vi "Task Scheduler Test.vi"() -> ()   [LabVIEW 2015]
uses:
  Re-use Libraries/Minimal Actor Framework/Actors/Base Actor/Actor/Common Config.ctl
  Re-use Libraries/Minimal Actor Framework/Actors/Base Actor/Actor/Front Panel State.ctl
  Re-use Libraries/Minimal Actor Framework/Messaging/Messenger/Messenger.lvclass
  Globals.vi
  Actors/Task Scheduler/API/Task Scheduler Actor API.lvclass
  Re-use Libraries/Minimal Actor Framework/Actors/Base Actor/Actor/Actor.lvclass
  Actors/Task Scheduler/Actor/Task Scheduler Actor.lvclass
panel:
  in  "Log Name":string
  in  "Period 2":dbl
  in  "Period":dbl
  in  "Data Logging":bool
  in  "Heartbeat":bool
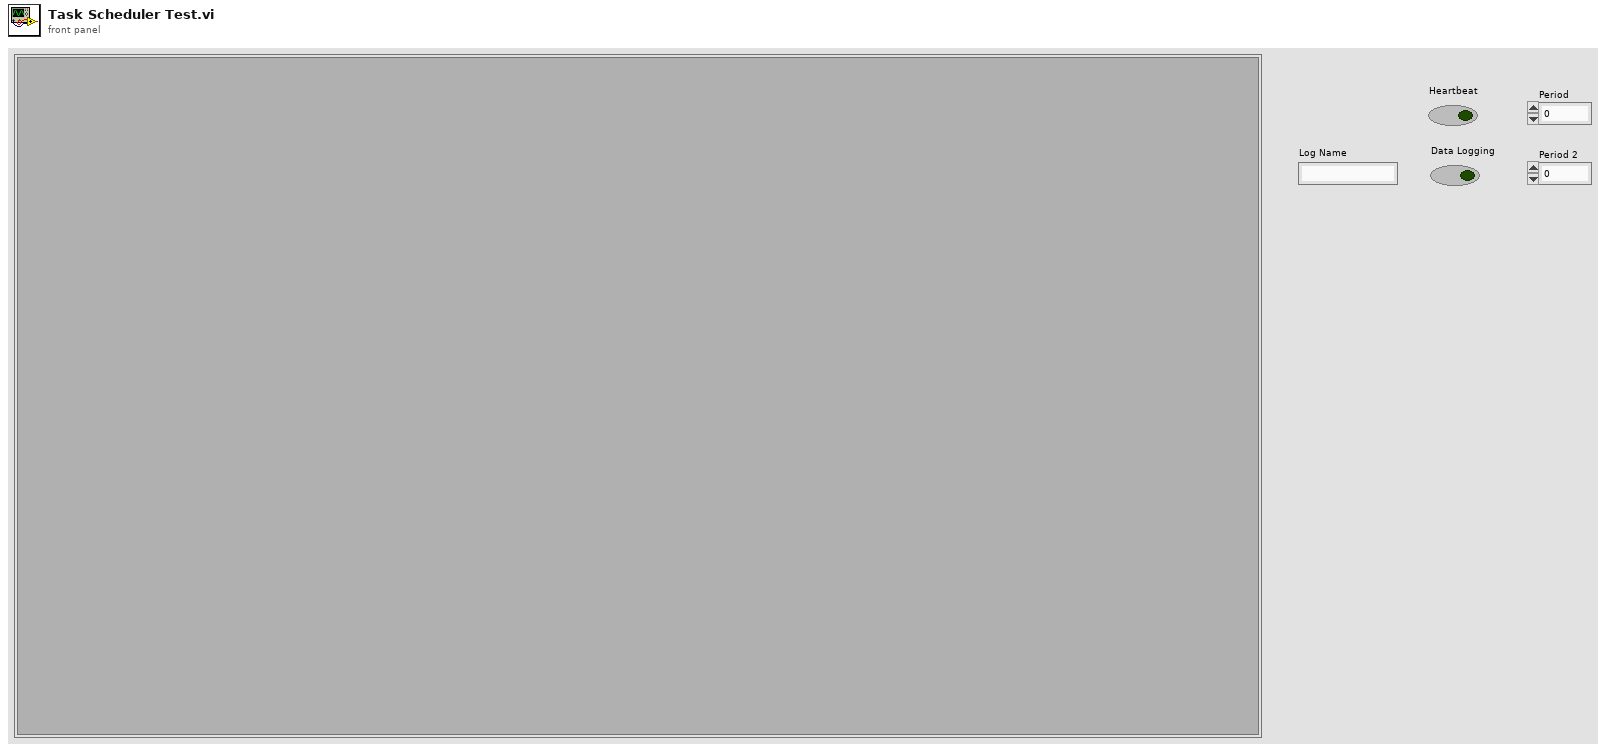
[diagram p1: front panel]
types:
  T1 = typedef "Actor.lvclass/Front Panel State.ctl" = enum32{"Invalid", "Standard", "Closed", "Hidden", "Minimized", "Maximized"}
  T2 = typedef "Actor.lvclass/Common Config.ctl" = cluster{"Launch Timeout [ms]":i32, "Wait For Launch Completed":bool, "Front Panel State":T1, "Close FP On Shutdown":bool, "Response Channel":refnum<class "Messenger.lvclass">, "Sub Panel":refnum<vi>}
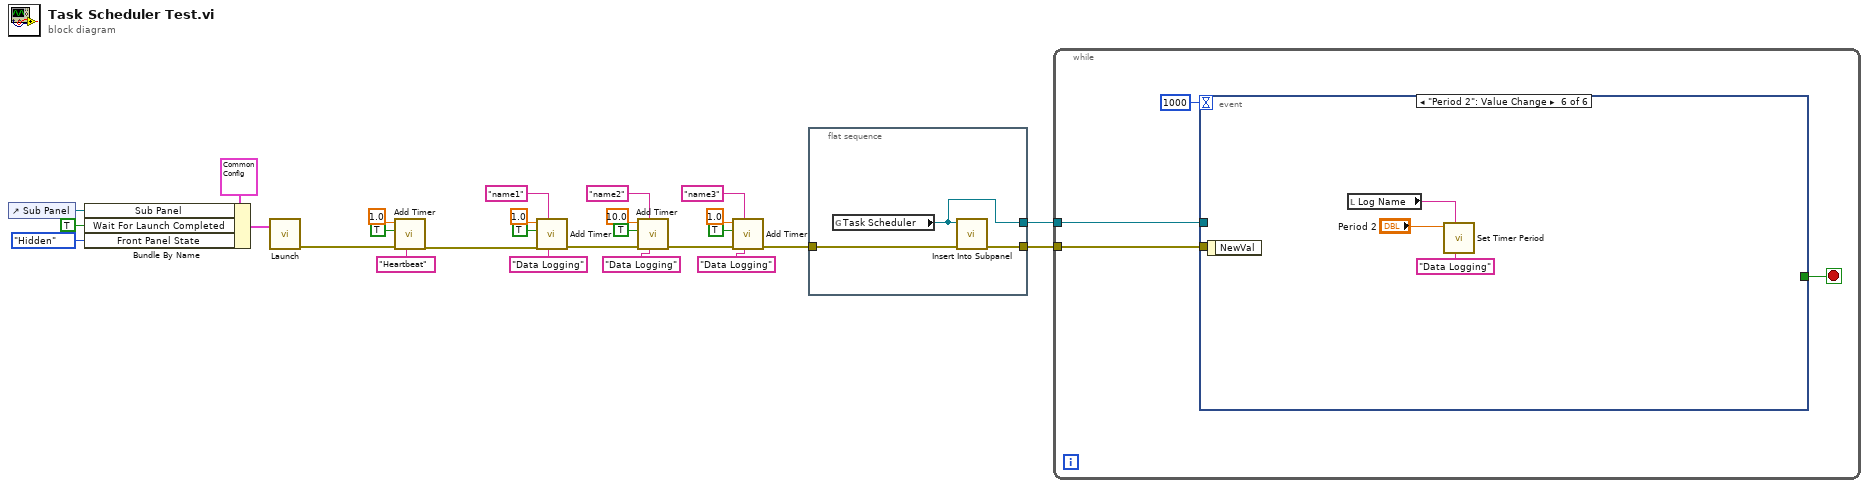
[diagram p0: block diagram]
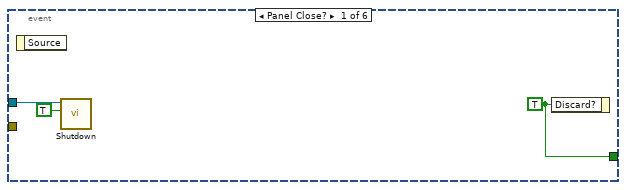
[diagram p2: hidden frame]
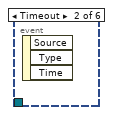
[diagram p3: hidden frame]
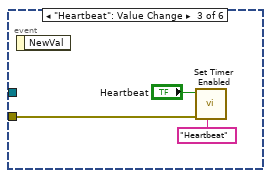
[diagram p4: hidden frame]
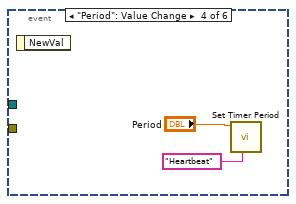
[diagram p5: hidden frame]
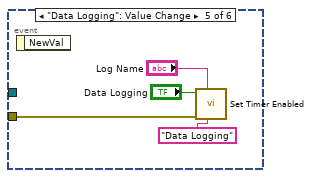
[diagram p6: hidden frame]
diagram:
  n1 = control-ref of="Sub Panel"() -> (w25:refnum<vi>)
  n2 = Bundle By Name(cluster=T2 {"Launch Timeout [ms]"=-1, "Wait For Launch Completed"=FALSE, "Front Panel State"=enum."Standard", "Close FP On Shutdown"=TRUE, "Response Channel"=refnum, "Sub Panel"=refnum} ("Common Config"), "Sub Panel"=w25, "Wait For Launch Completed"=TRUE, "Front Panel State"=Front_Panel_State."Hidden") -> (w26:T2)
  n3 = call "Launch.vi"("Common Config"=w26) -> ("error out"=w20:errorcluster)  [unwired: 9 in, 1 out]
  n4 = call "Add Timer.vi"("Name"="Heartbeat", "error in (no error)"=w20, "Enabled (T)"=TRUE ("Enabled"), "Period (1) [s]"=1.0 ("Period [s]")) -> ("error out"=w16:errorcluster)  [unwired: 7 in]
  n5 = call "Add Timer.vi"("Name"="Data Logging", "Metadata"="name1", "error in (no error)"=w16, "Enabled (T)"=TRUE ("Enabled"), "Period (1) [s]"=1.0 ("Period [s]")) -> ("error out"=w6:errorcluster)  [unwired: 6 in]
  n6 = call "Add Timer.vi"("Name"="Data Logging", "Metadata"="name2", "error in (no error)"=w6, "Enabled (T)"=TRUE ("Enabled"), "Period (1) [s]"=10.0 ("Period [s]")) -> ("error out"=w1:errorcluster)  [unwired: 6 in]
  n7 = call "Add Timer.vi"("Name"="Data Logging", "Metadata"="name3", "error in (no error)"=w1, "Enabled (T)"=TRUE ("Enabled"), "Period (1) [s]"=1.0 ("Period [s]")) -> ("error out"=w15:errorcluster)  [unwired: 6 in]
  n8 = flat-sequence {
    tunnel: w15 -> [w30]
    tunnel: [w29] -> w24
    tunnel: [w28] -> w23
    frame #0 {
      n9 = global read "Globals.vi" "Task Scheduler"() -> (w28:refnum<class "Task Scheduler Actor API.lvclass">)
      n10 = call-dynamic "Insert Into Subpanel.vi"("error in (no error)"=w30, "Actor API in"=w28) -> ("error out"=w29:errorcluster)  [unwired: 9 in]
    }
  }
  n11 = while {
    tunnel: w24 -> [w32]
    tunnel: w23 -> [w31]
    stop <- w34 stop-if-true
    n12 = event shown="[5] \"Period 2\": Value Change" {
      selector: _ -> [_ _ _ _ _ _]
      dyn-events: _ -> [_ _ _ _ _ _]
      timeout: 1000 -> [_ _ _ _ _ _]
      tunnel: [w37 _ _ _ _ _] -> w34
      tunnel: w32 -> [_ _ w40 _ w46 _]
      tunnel: w31 -> [w35 _ _ _ _ _]
      event Panel Close? {
        w37 = TRUE ("Discard?")
        n13 = event-data() -> ()  [unwired: 1 in, 1 out]
        n14 = call-dynamic "Shutdown.vi"("Wait For Shutdown (F)"=TRUE, "Actor API in"=w35) -> ()  [unwired: 9 in, 1 out]
        n15 = event-data("Discard?"=w37) -> ()  [unwired: 1 in, 1 out]
      }
      event Timeout {
        n16 = event-data() -> ()  [unwired: 1 in, 3 out]
      }
      event "Heartbeat": Value Change {
        n17 = event-data() -> ()  [unwired: 1 in, 1 out]
        n18 = call "Set Timer Enabled.vi"("Name"="Heartbeat", "error in (no error)"=w40, "Enabled (T)"="Heartbeat") -> ()  [unwired: 8 in, 1 out]
      }
      event "Period": Value Change {
        n19 = event-data() -> ()  [unwired: 1 in, 1 out]
        n20 = call "Set Timer Period.vi"("Name"="Heartbeat", "Period [s]"="Period") -> ()  [unwired: 9 in, 1 out]
      }
      event "Data Logging": Value Change {
        n21 = event-data() -> ()  [unwired: 1 in, 1 out]
        n22 = call "Set Timer Enabled.vi"("Name"="Data Logging", "Metadata"="Log Name", "error in (no error)"=w46, "Enabled (T)"="Data Logging") -> ()  [unwired: 7 in, 1 out]
      }
      event "Period 2": Value Change {
        n23 = event-data() -> ()  [unwired: 1 in, 1 out]
        n24 = local read "Log Name"() -> (w47:string)
        n25 = call "Set Timer Period.vi"("Name"="Data Logging", "Metadata"=w47, "Period [s]"="Period 2") -> ()  [unwired: 8 in, 1 out]
      }
    }
  }
